vi "atan2.vi"(1 "x":dbl, 2 "y":dbl) -> (0 "atan2":dbl)   [LabVIEW 2015]
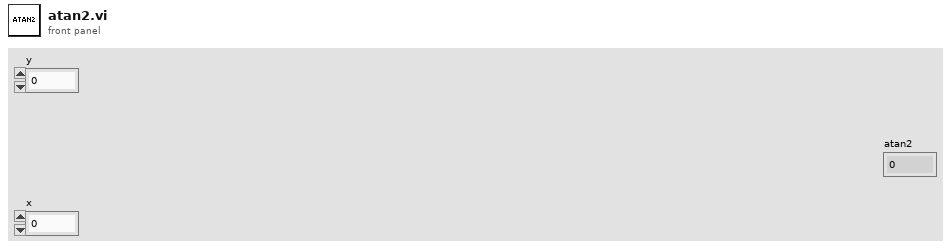
[diagram p1: front panel]
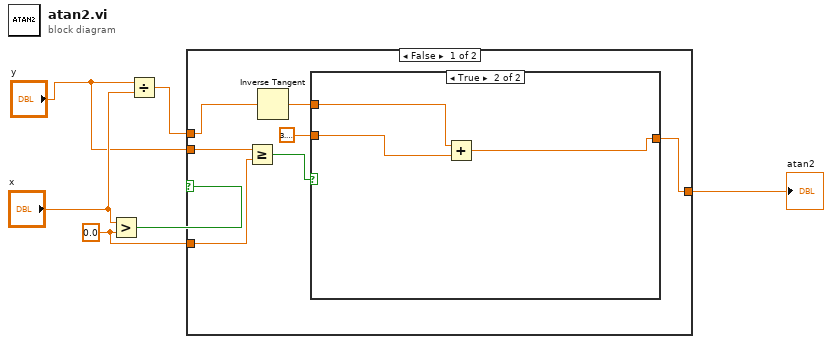
[diagram p0: block diagram]
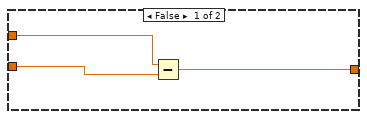
[diagram p2: hidden frame]
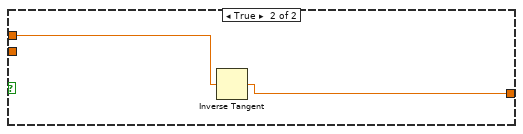
[diagram p3: hidden frame]
diagram:
  w2 = 0.0 ("y")
  n1 = Greater?(x="x", y=w2) -> (0:w6:bool)
  n2 = Divide(x="y", y="x") -> (x/y=w4:dbl)
  n3 = case shown="False" w6 {
    tunnel: w4 -> [w11 w21]
    tunnel: [w7 w20] -> w3
    tunnel: w2 -> [w13 _]
    tunnel: "y" -> [w10 _]
    frame False {
      n4 = Greater Or Equal?(x=w10, y=w13) -> (x >= y?=w12:bool)
      n5 = Inverse Tangent(1:w11) -> (0:w9:dbl)
      n6 = case shown="True" w12 {
        tunnel: w9 -> [w16 w19]
        tunnel: 3.141592653589793 -> [w15 w18]
        tunnel: [w14 w17] -> w7
        frame False {
          n7 = Subtract(x=w16, y=w15) -> (x-y=w14:dbl)
        }
        frame True {
          n8 = Add(x=w19, y=w18) -> (x+y=w17:dbl)
        }
      }
    }
    frame True {
      n9 = Inverse Tangent(1:w21) -> (0:w20:dbl)
    }
  }
  "atan2" <- w3
